vi "ParseConfigText.vi"(8 "error in (no error)":errorcluster, 11 "InstrumentConfig(ini)":string) -> (0 "error out":errorcluster, 3 "Instruments":T1[](array[typedef]))   [LabVIEW 2020, in "VdInstrument.lvclass"]
uses:
  VdInstrument.lvclass
  InstrumentConfig.ctl
  InstrumentType.ctl
  <vilib>/Utility/config.llb/Read Key (String).vi
  <vilib>/Utility/config.llb/NI_LVConfig.lvlib
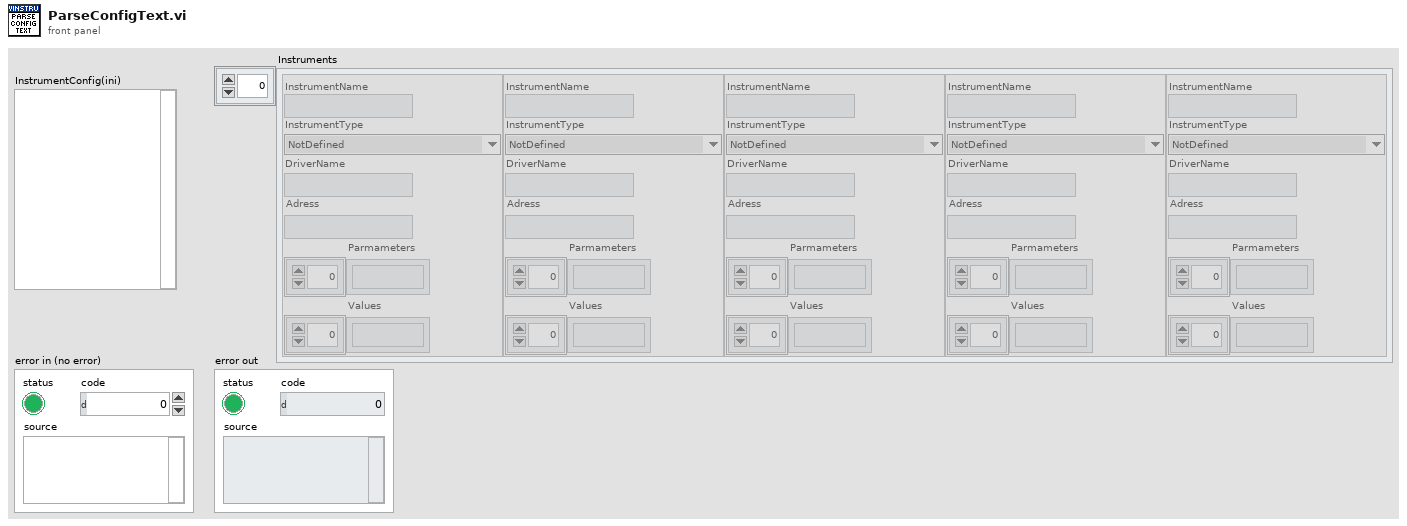
[diagram p1: front panel]
types:
  T1 = typedef "VdInstrument.lvclass/InstrumentConfig.ctl" = cluster{"InstrumentName":string, "InstrumentType":T2, "DriverName":string, "Adress":string, "Parmameters":string[], "Values":string[]}
  T2 = typedef "VdInstrument.lvclass/InstrumentType.ctl" = enum16{"NotDefined", "AirflowController", "AnalogInput", "AnalogOutput", "AutoCollimator", "BeamProfiler", "DMM", "DigitalControl", "DigitalInput", "DisplacementSensor", "Encoder", "ForceSensor", "FrequencyCounter", "FunctionGenerator", "GelDispensingRobot", "GlueDispenser", "Hexapod", "IRCamera", "ImageGenerator", "LabelPrinter", "LightController", "LightIndicator", "Load", "Multimeter", "OpticalAttenuatorPowerMeter", "OpticalChannelMonitor", "OpticalLaser", "OpticalPolarizationController", "OpticalPowerAttenuator", "OpticalPowerMeter", "OpticalSpectrumAnalyzer", "PDLMeter", "PolarisationScrambler", "PolarizationAnalyzer", "PositionSensitiveDetector", "PowerSupply", "PressureController", "Robot", "SLRCamera", "ScrewdriverController", "SignalAnalyzer", "SignalGenerator", "SixAxisStage", "SolderingStation", "SpectrumAnalyzer", "StepperMotor", "Stirrer", "SweptWavelengthSystem", "Switch", "TemperatureChamber", "TemperatureController", "TemperatureSensor", "TunableLaser", "UVCuring", "UsbHub", "VisionCamera", "WavelengthMeter", "WeldingLaser"}
  T3 = typedef "NI_LVConfig.lvlib/Config Data RefNum.ctl" = refnum<k1>
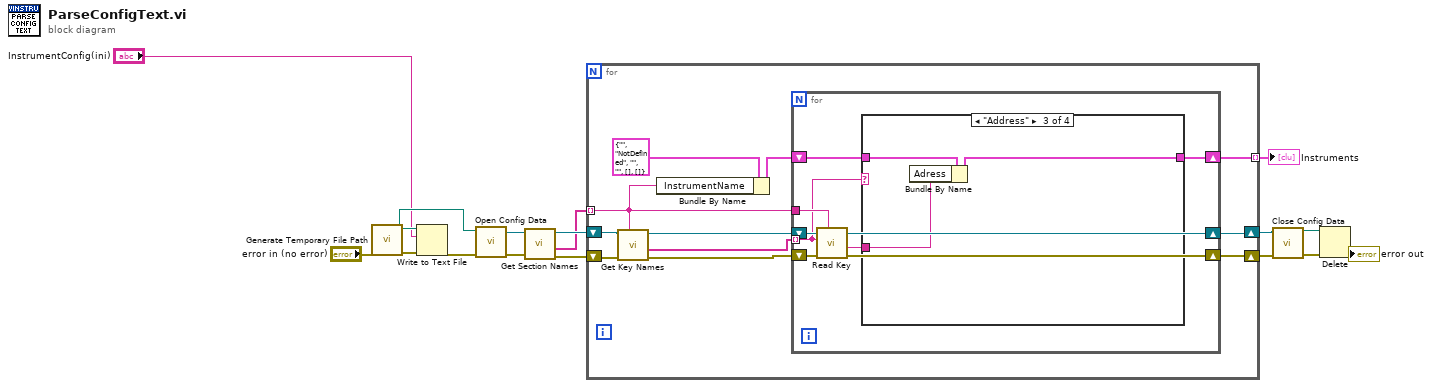
[diagram p0: block diagram]
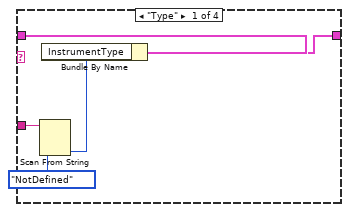
[diagram p2: hidden frame]
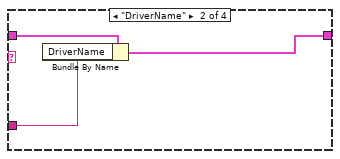
[diagram p3: hidden frame]
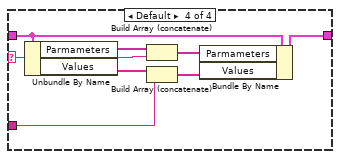
[diagram p4: hidden frame]
diagram:
  n1 = call <vilib>:"Generate Temporary File Path.vi"("error in (no error)"="error in (no error)") -> ("error out"=w4:errorcluster, "Unique Temporary File Path"=w5:path)  [unwired: 9 in]
  n2 = Write to Text File(file (use dialog)=w5, text="InstrumentConfig(ini)", error in=w4) -> (error out=w6:errorcluster)  [unwired: 1 in, 2 out]
  n3 = call <vilib>:"Open Config Data.vi"("error in (no error)"=w6, "configuration file path"=w5) -> ("error out"=w7:errorcluster, "refnum"=w8:T3)  [unwired: 7 in, 1 out]
  n4 = call <vilib>:"Get Section Names.vi"("error in (no error)"=w7, "refnum"=w8) -> ("error out"=w9:errorcluster, "section names"=w10:string[], "refnum out"=w11:T3)  [unwired: 7 in]
  n5 = for {
    tunnel: w10 -> [w17] mode=indexing
    shift-right: [w20] -> w13
    shift-left: w11 -> [w26]
    shift-right: [w21] -> w12
    shift-left: w9 -> [w27]
    tunnel: [w19] -> w1 mode=indexing
    n6 = call <vilib>:"Get Key Names.vi"("section"=w17, "error in (no error)"=w27, "refnum"=w26) -> ("error out"=w24:errorcluster, "key names"=w23:string[], "refnum out"=w25:T3)  [unwired: 5 in, 1 out]
    n7 = Bundle By Name(cluster=T1 {"InstrumentName"="", "InstrumentType"=enum."NotDefined", "DriverName"="", "Adress"="", "Parmameters"=[], "Values"=[]} ("InstrumentConfig"), "InstrumentName"=w17) -> (w18:T1)
    n8 = for {
      tunnel: w17 -> [w34]
      tunnel: w23 -> [w28] mode=indexing
      shift-right: [w31] -> w19
      shift-left: w18 -> [w32]
      shift-right: [w30] -> w21
      shift-left: w24 -> [w35]
      shift-right: [w29] -> w20
      shift-left: w25 -> [w36]
      n9 = call-poly <vilib>:"Read Key.vi"("section"=w34, "error in (no error)"=w35, "key"=w28, "refnum"=w36) -> ("error out"=w30:errorcluster, "value"=w33:string, "refnum out"=w29:T3)  [unwired: 4 in, 1 out]
      n10 = case shown="\"Address\"" w28 {
        selector: w28 -> [_ _ _ w53]
        tunnel: w33 -> [w41 w42 w45 w48]
        tunnel: w32 -> [w39 w44 w47 w51]
        tunnel: [w37 w43 w46 w55] -> w31
        frame "Type" {
          n11 = Scan From String(input string=w41, default 1=InstrumentType."NotDefined" ("InstrumentType")) -> (output 1=w38:T2)  [unwired: 3 in, 3 out]
          n12 = Bundle By Name(cluster=w39, "InstrumentType"=w38) -> (w37:T1)
        }
        frame "DriverName" {
          n13 = Bundle By Name(cluster=w44, "DriverName"=w42) -> (w43:T1)
        }
        frame "Address" {
          n14 = Bundle By Name(cluster=w47, "Adress"=w45) -> (w46:T1)
        }
        frame Default {
          n15 = Unbundle By Name(w51) -> ("Parmameters"=w54:string[], "Values"=w50:string[])
          n16 = Build Array (concatenate)(w54, w53) -> (w52:string[])
          n17 = Build Array (concatenate)(w50, w48) -> (w49:string[])
          n18 = Bundle By Name(cluster=w51, "Parmameters"=w52, "Values"=w49) -> (w55:T1)
        }
      }
    }
  }
  "Instruments" <- w1
  n19 = call <vilib>:"Close Config Data.vi"("error in (no error)"=w12, "refnum"=w13) -> ("error out"=w15:errorcluster, "file path"=w14:path)  [unwired: 8 in]
  n20 = Delete(path (use dialog)=w14, error in=w15) -> (error out=→"error out":errorcluster)  [unwired: 3 in, 2 out]
